vi "sm.vi"(2 "c":bool, 3 "b":bool, 4 "a":bool) -> (0 "C":bool, 1 "S":bool)   [LabVIEW 2013]
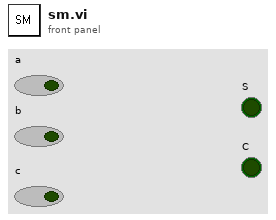
[diagram p1: front panel]
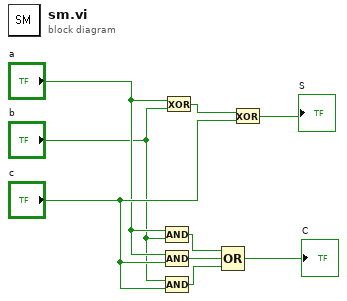
[diagram p0: block diagram]
diagram:
  n1 = Exclusive Or(1:"b", 2:"a") -> (0:w9:bool)
  n2 = Compound Arithmetic op=AND("a", "b") -> (w6:bool)
  n3 = Compound Arithmetic op=AND("a", "c") -> (w5:bool)
  n4 = Compound Arithmetic op=AND("b", "c") -> (w4:bool)
  n5 = Compound Arithmetic op=OR(w6, w5, w4) -> (→"C":bool)
  n6 = Exclusive Or(1:"c", 2:w9) -> (0:→"S":bool)
